vi "Act 19.vi"() -> ()   [LabVIEW 2010]
uses:
  act/lv_07/lv_07.lvlib
panel:
  out "Te (en mois)":dbl
  in  "Cc":dbl=20.0
  in  "T":dbl=0.15
  out "error out":errorcluster caption="err out"
  in  "err in":errorcluster
  out "Qe":dbl
  in  "Pu":dbl
  in  "Qa":dbl
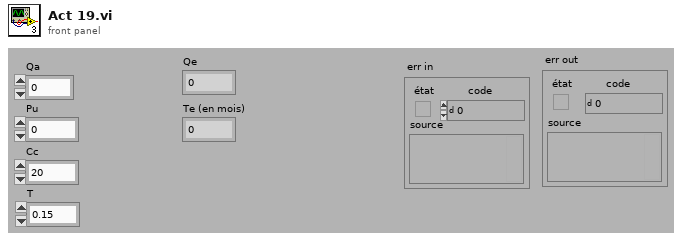
[diagram p1: front panel]
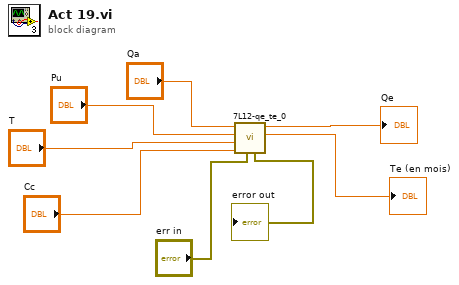
[diagram p0: block diagram]
diagram:
  n1 = call "7L12-qe_te_0.vi"("err in"="err in", "Cc"="Cc", "T"="T", "Pu"="Pu", "Qa"="Qa") -> ("Te (en mois)"=→"Te (en mois)":dbl, "Qe"=→"Qe":dbl, "error out"=→"error out":errorcluster)  [unwired: 4 in]
